vi "Apply_Parent_Settings.vi"(8 "error in (no error)":errorcluster, 10 "sourceItems in":refnum<class "AB_Source.lvclass">[](array[class]), 11 "AB_Source_Library in":refnum<class "AB_Source_Library.lvclass">) -> (0 "error out":errorcluster, 1 "parentApplies":T1, 2 "sourceItems out":refnum<class "AB_Source.lvclass">[](array[class]), 3 "AB_Source_Library out":refnum<class "AB_Source_Library.lvclass">)   [LabVIEW 2020, in "AB_Source_Library.lvclass"]
uses:
  <vilib>/AppBuilder/AB_Classes/Source/Library/AB_Source_Library.lvclass
  <vilib>/AppBuilder/AB_Parent_Applies.ctl
  <vilib>/AppBuilder/AB_Classes/Source/AB_Source.lvclass
  e:/builds/penguin/labview/branches/2020/dev/dist/vi.lib/AppBuilder/AB_Classes/Source/AB_Source.lvclass
  <vilib>/AppBuilder/AB_Classes/Source/Library/AB_Source_Library.lvclass/AB_Source_Library.ctl
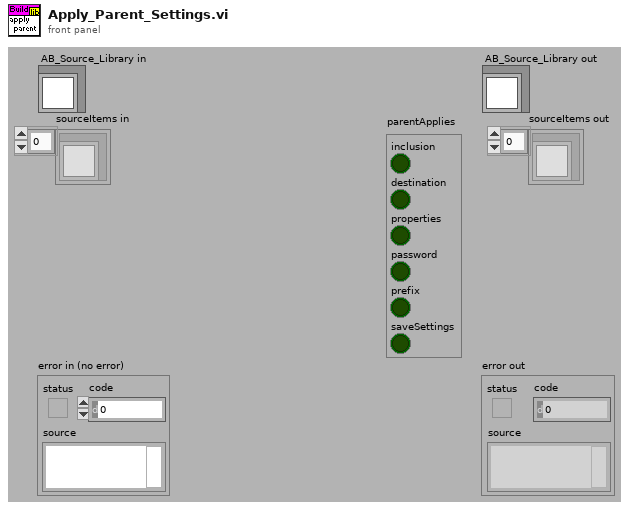
[diagram p1: front panel]
types:
  T1 = typedef "AB_Parent_Applies.ctl" = cluster{"inclusion":bool, "destination":bool, "properties":bool, "password":bool, "prefix":bool, "saveSettings":bool}
  T2 = typedef "AB_Source.ctl" = cluster{"path":path, "itemID":string, "parentIndex":i32, "sourceInclusion":T3, "destinationIndex":i32, "properties":T4[], "newName":string, "lvfile":bool, "valid":bool, "eng_inBuild":bool, "eng_isNonVILink":bool, "Amalgamation":bool, "Amalgamation Piece":bool, "eng_delimitedName":string, "preventRename":bool}
  T3 = typedef "AB_Source_Inclusion.ctl" = enum16{"IncludeIfReferenced", "Include", "Exclude", "TopLevel"}
  T4 = typedef "AB_Source_Properties.ctl" = cluster{"sourcePropertyType":T5, "value":variant}
  T5 = typedef "AB_Source_Property_Type.ctl" = enum16{"Remove block diagram", "Remove front panel", "Password", "Window has title bar", "Show menu bar", "Show vertical scroll bar", "Show horizontal scroll bar", "Show toolbar", "Show Abort button", "Show fp when called", "Window behavior", "Allow user to close window", "Window run-time position", "Run when opened", "Allow debugging", "Auto error handling", "Generate guard code", "Use stack variables", "Expression folding", "Integer only", "Inline subVI"}
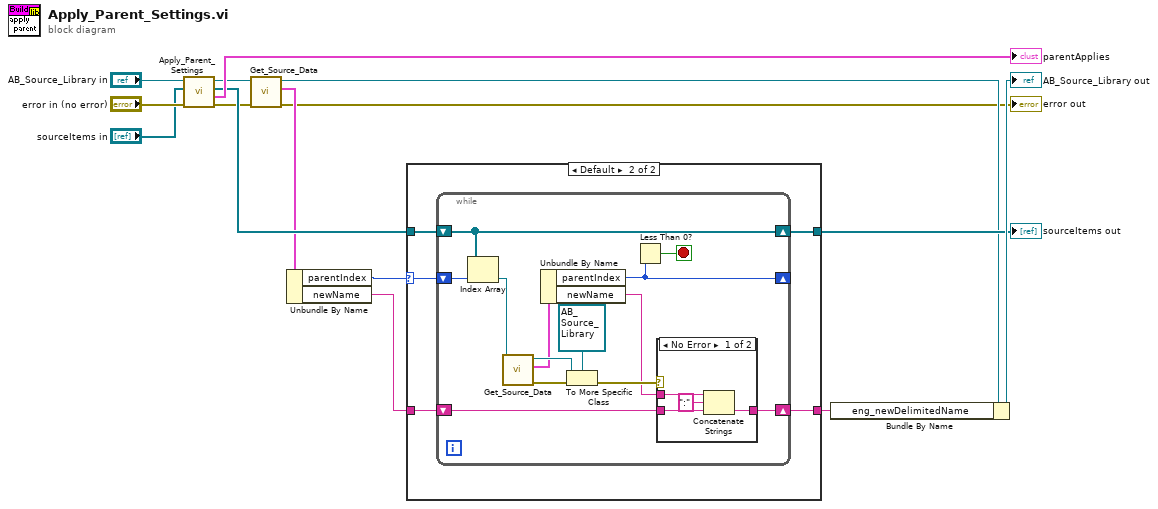
[diagram p0: block diagram]
diagram:
  n1 = call-parent "Apply_Parent_Settings.vi"("error in (no error)"="error in (no error)", "sourceItems in"="sourceItems in", "AB_Source in"="AB_Source_Library in") -> ("error out"=w2:errorcluster, "parentApplies"=→"parentApplies":T1, "sourceItems out"=w9:refnum<class "AB_Source.lvclass">[], "AB_Source out"=w7:refnum<class "AB_Source_Library.lvclass">)  [unwired: 5 in]
  n2 = call <vilib>:"Get_Source_Data.vi"("error in (no error)"=w2, "Class in"=w7) -> ("error out"=→"error out":errorcluster, "data"=w6:T2, "Class out"=w3:refnum<class "AB_Source_Library.lvclass">)  [unwired: 7 in]
  n3 = Unbundle By Name(w6) -> ("parentIndex"=w5:i32, "newName"=w4:string)
  n4 = case shown="Default" w5 {
    selector: w5 -> [_ w22]
    tunnel: w9 -> [w16 w21]
    tunnel: w4 -> [w17 w20]
    tunnel: [w17 w19] -> w10
    tunnel: [w16 w18] -> w8
    frame -1 {
    }
    frame Default {
      n5 = while {
        shift-right: [w24] -> _
        shift-left: w22 -> [w34]
        shift-right: [w35] -> w18
        shift-left: w21 -> [w35]
        shift-right: [w29] -> w19
        shift-left: w20 -> [w30]
        stop <- w33 stop-if-true
        n6 = Index Array(array=w35, index=w34) -> (element=w28:refnum<class "AB_Source.lvclass">)
        n7 = call <vilib>:"Get_Source_Data.vi"("Class in"=w28) -> ("error out"=w26:errorcluster, "data"=w25:T2, "Class out"=w27:refnum<class "AB_Source.lvclass">)  [unwired: 8 in]
        n8 = Unbundle By Name(w25) -> ("parentIndex"=w24:i32, "newName"=w23:string)
        n9 = To More Specific Class(target class=refnum<class "AB_Source_Library.lvclass"> refnum ("AB_Source_Library in"), reference=w27, error in=w26) -> (error out=w32:errorcluster)  [unwired: 1 out]
        n10 = Less Than 0?(x=w24) -> (x < 0?=w33:bool)
        n11 = case shown="No Error" w32 {
          tunnel: w30 -> [w38 w40]
          tunnel: [w37 w40] -> w29
          tunnel: w23 -> [w36 _]
          frame No Error {
            n12 = Concatenate Strings(w36, ":" ("string"), w38) -> (w37:string)
          }
          frame Error {
          }
        }
      }
    }
  }
  "sourceItems out" <- w8
  n13 = Bundle By Name(cluster=w3, "eng_newDelimitedName"=w10) -> (→"AB_Source_Library out":refnum<class "AB_Source_Library.lvclass">)
